vi "Initialize.vi"(4 "id":string, 6 "Transform":string, 8 "error in (no error)":errorcluster, 9 "Style":string, 10 "rect":T1, 11 "Rectangle in":refnum<class "Rectangle.lvclass">) -> (0 "error out":errorcluster, 3 "Rectangle out":refnum<class "Rectangle.lvclass">)   [LabVIEW 2019, in "Rectangle.lvclass"]
uses:
  Rectangle.lvclass
  InitializeInformation.ctl
  TransformTokenizer/TransformTokenizer.lvclass
  CSSProperties/CSSProperties.lvclass
  Rectangle.lvclass/Rectangle.ctl
  TransformTokenizer/TransformTokenizer.lvclass/TransformTokenizer.ctl
  Transform/Transform.lvclass
  Transform.Matrix/Transform.Matrix.lvclass
  C:/Users/Albro/Documents/GitHub/AFM-Lithography/lvsrc/Classes/Parse/Transform/Transform.lvclass
  Transform.Translate/Transform.Translate.lvclass
  Transform.Rotate/Transform.Rotate.lvclass
  Transform.Skew/Transform.Skew.lvclass
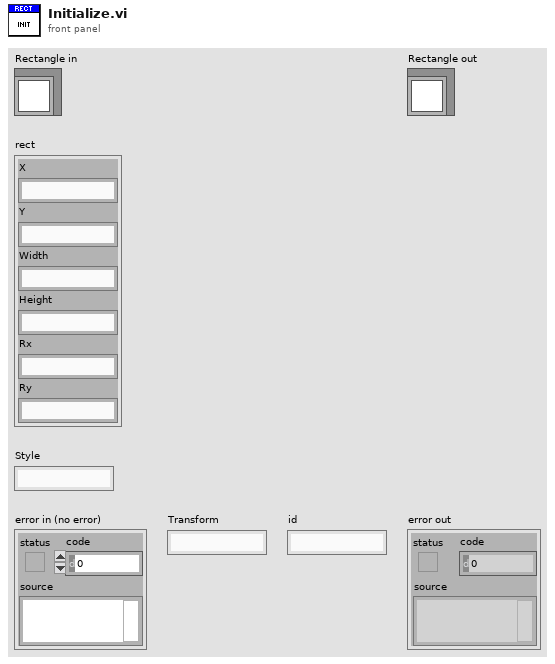
[diagram p1: front panel]
types:
  T1 = typedef "Rectangle.lvclass/InitializeInformation.ctl" = cluster{"X":string, "Y":string, "Width":string, "Height":string, "Rx":string, "Ry":string}
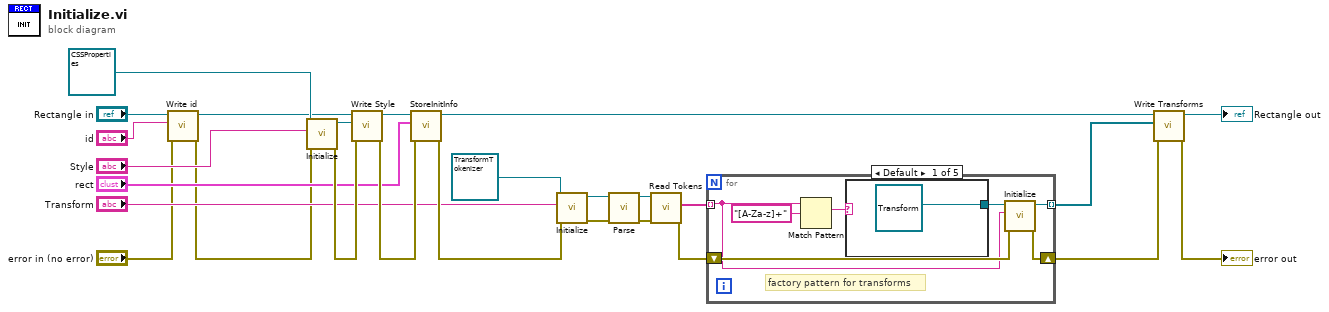
[diagram p0: block diagram]
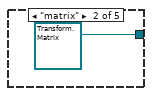
[diagram p2: hidden frame]
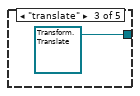
[diagram p3: hidden frame]
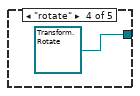
[diagram p4: hidden frame]
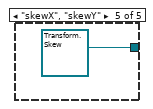
[diagram p5: hidden frame]
diagram:
  n1 = call-dynamic "Write id.vi"("error in (no error)"="error in (no error)", "id"="id", "SVG Object in"="Rectangle in") -> ("error out"=w1:errorcluster, "SVG Object out"=w4:refnum<class "Rectangle.lvclass">)  [unwired: 7 in]
  n2 = call "Initialize.vi"("error in (no error)"=w1, "Properties String"="Style", "CSSProperties in"=refnum<class "CSSProperties.lvclass"> refnum) -> ("error out"=w19:errorcluster, "CSSProperties out"=w7:refnum<class "CSSProperties.lvclass">)  [unwired: 7 in]
  n3 = call "Write Style.vi"("error in (no error)"=w19, "CSSProperties.lvclass"=w7, "Rectangle in"=w4) -> ("error out"=w20:errorcluster, "Rectangle out"=w12:refnum<class "Rectangle.lvclass">)  [unwired: 7 in]
  n4 = call "StoreInitInfo.vi"("error in (no error)"=w20, "rect"="rect", "Rectangle in"=w12) -> ("error out"=w23:errorcluster, "Rectangle out"=w11:refnum<class "Rectangle.lvclass">)  [unwired: 7 in]
  n5 = call "Initialize.vi"("error in (no error)"=w23, "Transform Attribute String"="Transform", "TransformTokenizer in"=refnum<class "TransformTokenizer.lvclass"> refnum) -> ("error out"=w26:errorcluster, "TransformTokenizer out"=w18:refnum<class "TransformTokenizer.lvclass">)  [unwired: 7 in]
  n6 = call "Parse.vi"("error in (no error)"=w26, "TransformTokenizer in"=w18) -> ("error out"=w25:errorcluster, "TransformTokenizer out"=w16:refnum<class "TransformTokenizer.lvclass">)  [unwired: 8 in]
  n7 = call "Read Tokens.vi"("error in (no error)"=w25, "TransformTokenizer in"=w16) -> ("error out"=w24:errorcluster, "Transforms"=w15:string[])  [unwired: 7 in, 1 out]
  n8 = for {
    tunnel: w15 -> [w27] mode=indexing
    shift-right: [w32] -> w22
    shift-left: w24 -> [w33]
    tunnel: [w28] -> w9 mode=indexing
    # "factory pattern for transforms"
    n9 = Match Pattern(string=w27, regular expression="[A-Za-z]+") -> (match substring=w30:string)  [unwired: 1 in, 3 out]
    n10 = case shown="Default" w30 {
      tunnel: [refnum<class "Transform.lvclass"> refnum ("Transform in") refnum<class "Transform.Matrix.lvclass"> refnum ("Transform.Matrix.lvclass") refnum<class "Transform.Translate.lvclass"> refnum ("Transform.Translate.lvclass") refnum<class "Transform.Rotate.lvclass"> refnum ("Transform.Rotate.lvclass") refnum<class "Transform.Skew.lvclass"> refnum ("Transform.Skew.lvclass")] -> w29
      frame Default {
      }
      frame "matrix" {
      }
      frame "translate" {
      }
      frame "rotate" {
      }
      frame "skewX", "skewY" {
      }
    }
    n11 = call-dynamic "Initialize.vi"("error in (no error)"=w33, "Transform"=w27, "Transform in"=w29) -> ("error out"=w32:errorcluster, "Transform out"=w28:refnum<class "Transform.lvclass">)  [unwired: 7 in]
  }
  n12 = call "Write Transforms.vi"("error in (no error)"=w22, "Transforms"=w9, "Rectangle in"=w11) -> ("error out"=→"error out":errorcluster, "Rectangle out"=→"Rectangle out":refnum<class "Rectangle.lvclass">)  [unwired: 7 in]
